vi "Hardware - NI 9411-2 (Digital Input) Host.vi"() -> ()   [LabVIEW 2015, in "ECS-Host.lvlib"]
uses:
  ECS-Host.lvlib
panel:
  out "FPGAWriteError":bool
  out "FPGAReadError":bool
  in  "DigitalInvertConfig":u32
  out "DigitalInputBooleanArray":u32
  out "_Channel Names":string[](array[string])
  out "Freq":sgl[](array[numeric]) format="%#_5f"
  out "DC":sgl[](array[numeric]) step=0.1 format="%.2f"
  out "PulseWidth":sgl[](array[numeric]) step=0.1 format="%#_5f"
  in  "_Digital_InvertConfig_Array":bool[](array[boolean])=[FALSE, FALSE, FALSE, FALSE, FALSE, FALSE, FALSE, FALSE, FALSE, FALSE, FALSE, FALSE, FALSE, FALSE, FALSE, FALSE, FALSE, FALSE, FALSE, FALSE, FALSE, FALSE, FALSE, FALSE, FALSE, FALSE, FALSE, FALSE, FALSE, FALSE, FALSE, FALSE]
  in  "DigitalFilt":sgl[](array[numeric]) format="%#.2f"
  out "_9411_DigInput_Array":bool[](array[boolean])
  # "Note: By default, the wires for NI 9411 Digital Input Module Channel 0 through 2 are routed through a switching terminal block to allow user to select between a 2.5V pull-up for higher logic level threshold for Single-ended input mode or a b-pin pass through for Differential input mode."
  # "Channel Name"
  # "State"
  # "Freq [Hz]"
  # "DC [%]"
  # "PW [ms] [msec]"
  # "Invert Input"
  # "Filter [us]"
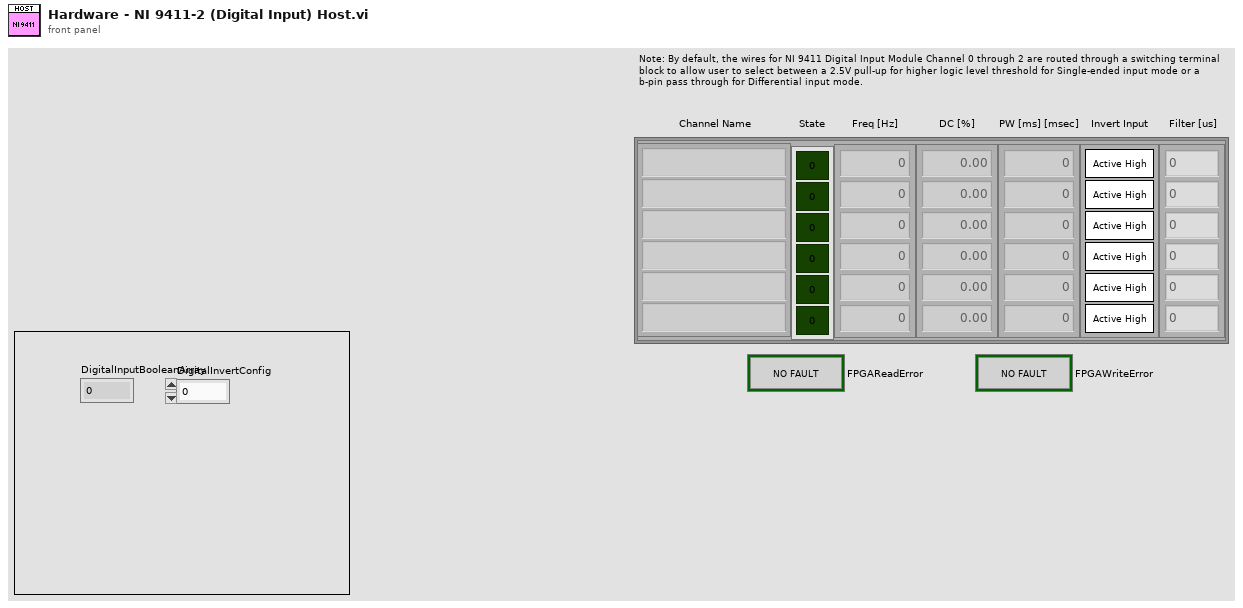
[diagram p1: front panel]
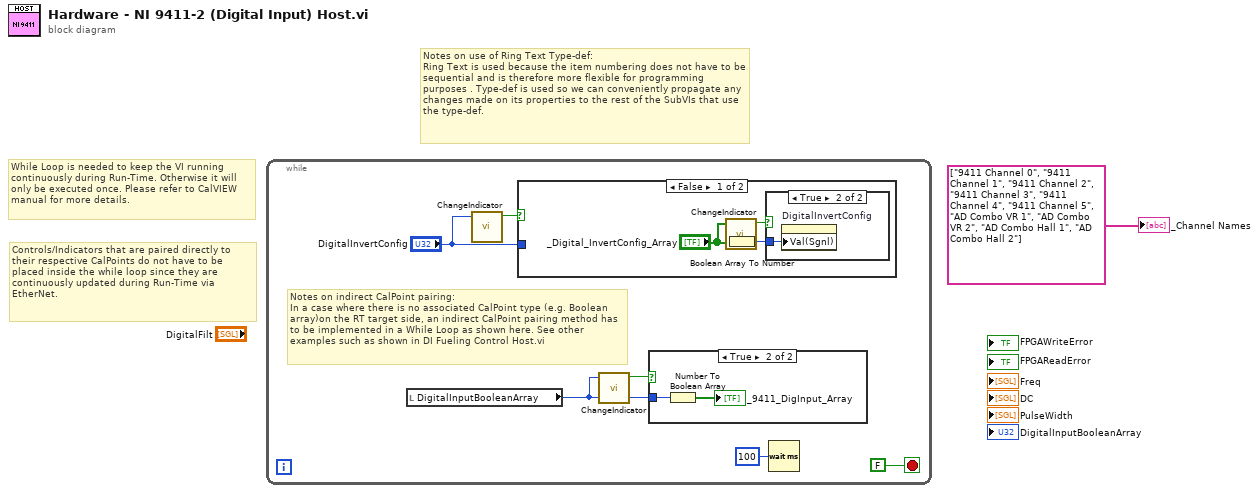
[diagram p0: block diagram]
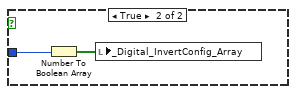
[diagram p3: hidden frame]
diagram:
  # "Notes on use of Ring Text Type-def:\nRing Text is used because the item numbering does not have to be sequential and is therefore more flexible for programming purposes . Type-def is used so we can conveniently propagate any changes made on its properties to the rest of the SubVIs that use the type-def."
  # "While Loop is needed to keep the VI running\ncontinuously during Run-Time. Otherwise it will only be executed once. Please refer to CalVIEW manual for more details."
  # "Controls/Indicators that are paired directly to their respective CalPoints do not have to be placed inside the while loop since they are continuously updated during Run-Time via EtherNet."
  n1 = while {
    stop <- FALSE stop-if-true
    # "Notes on indirect CalPoint pairing:\nIn a case where there is no associated CalPoint type (e.g. Boolean array)on the RT target side, an indirect CalPoint pairing method has to be implemented in a While Loop as shown here. See other examples such as shown in DI Fueling Control Host.vi"
    n2 = local read "DigitalInputBooleanArray"() -> (w5:u32)
    n3 = call "ChangeIndicator.vi"("Input"="DigitalInvertConfig") -> ("Change"=w3:bool)  [unwired: 9 in]
    n4 = case shown="False" w3 {
      tunnel: "DigitalInvertConfig" -> [_ w13]
      frame False {
        n5 = call "ChangeIndicator.vi"("Input"="_Digital_InvertConfig_Array") -> ("Change"=w9:bool)  [unwired: 9 in]
        n6 = Boolean Array To Number(Boolean array="_Digital_InvertConfig_Array") -> (number=w10:u32)
        n7 = case shown="True" w9 {
          tunnel: w10 -> [_ w11]
          frame False {
          }
          frame True {
            n8 = property on="DigitalInvertConfig" class="DigNum (strict)"("Val(Sgnl)"=w11) -> ()  [unwired: 2 in, 2 out]
          }
        }
      }
      frame True {
        n9 = Number To Boolean Array(number=w13) -> (Boolean array=w12:bool[])
        n10 = local write "_Digital_InvertConfig_Array"(w12) -> ()
      }
    }
    n11 = call "ChangeIndicator.vi"("Input"=w5) -> ("Change"=w4:bool)  [unwired: 9 in]
    n12 = case shown="True" w4 {
      tunnel: w5 -> [_ w14]
      frame False {
      }
      frame True {
        n13 = Number To Boolean Array(number=w14) -> (Boolean array=→"_9411_DigInput_Array":bool[])
      }
    }
    n14 = Wait (ms)(milliseconds to wait=u32 100) -> ()  [unwired: 1 out]
  }
  "_Channel Names" <- string[] ["9411 Channel 0", "9411 Channel 1", "9411 Channel 2", "9411 Channel 3", "9411 Channel 4", "9411 Channel 5", "AD Combo VR 1", "AD Combo VR 2", "AD Combo Hall 1", "AD Combo Hall 2"]
